vi "startup.vi"(8 "error in (no error)":errorcluster, 11 "AnalysisResultsViewer in":refnum<class "AnalysisResultsViewer.lvclass">) -> (0 "error out":errorcluster, 3 "AnalysisResultsViewer out":refnum<class "AnalysisResultsViewer.lvclass">)   [LabVIEW 2011, in "Views.lvlib" / "Camera.lvlib" / "AnalysisResultsViewer.lvclass"]
uses:
  AnalysisResultsViewer.lvclass
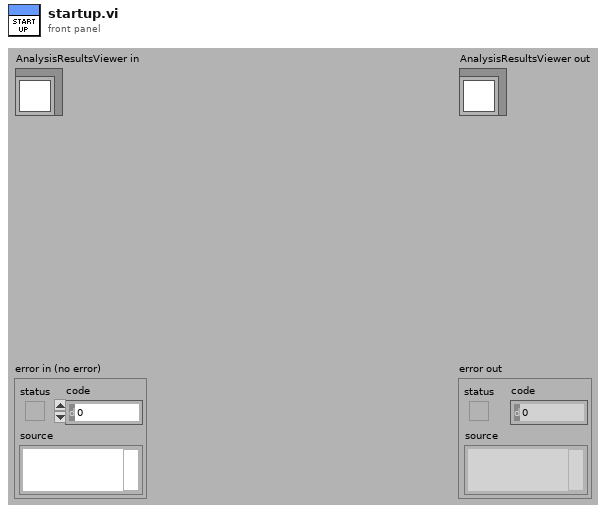
[diagram p1: front panel]
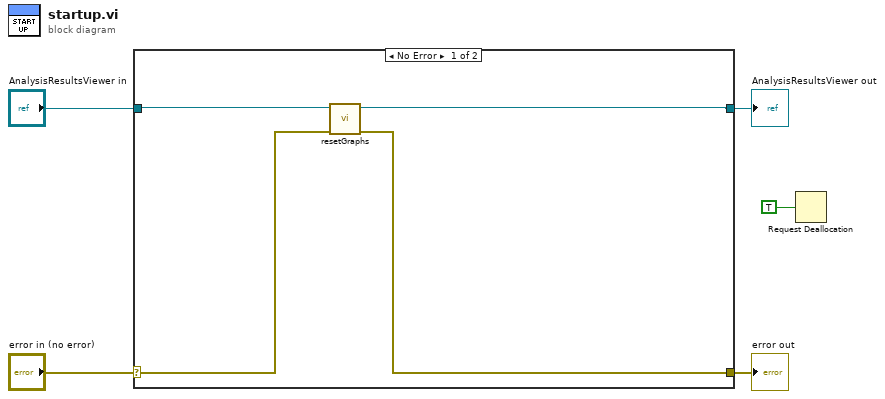
[diagram p0: block diagram]
diagram:
  n1 = case shown="No Error" "error in (no error)" {
    selector: "error in (no error)" -> [w7 w11]
    tunnel: [w6 w11] -> w4
    tunnel: [w8 w10] -> w2
    tunnel: "AnalysisResultsViewer in" -> [w9 w10]
    frame No Error {
      n2 = call "resetGraphs.vi"("error in (no error)"=w7, "AnalysisResultsViewer in"=w9) -> ("error out"=w6:errorcluster, "AnalysisResultsViewer out"=w8:refnum<class "AnalysisResultsViewer.lvclass">)  [unwired: 8 in]
    }
    frame Error {
    }
  }
  "error out" <- w4
  "AnalysisResultsViewer out" <- w2
  n3 = Request Deallocation(TRUE ("flag")) -> ()
